vi "Start!.vi"() -> ()   [LabVIEW 2015]
doc: "This VI is designed to launch the VIs needed to do data acquisition on the microscope in the required order. The VIs can be launched from the Glimpse library (used to launch Glimpse itself) or from the plug-ins library (used to launch the data acquisition plug-in and any hardware-control plug-ins that are needed). It is suggested that users modify settings as needed and save the modified version with a name descriptive of the type of experiment. (That's why this is a separate file, not included in the plug-ins library.) (Remember to right-click/Data Operations/Make current value default value so that your altered setting will be saved for the next time!)"
uses:
  h-nu-ixon/Start! globals.vi
  Microscope software version global.vi
  h-nu-ixon/Microscope ID global.vi
  Glimpse core/GLIMPSE Globals.vi
  ixon1024/HAL Camera specifications globals.vi
  h-nu-ixon/knob global.vi
  h-nu-ixon/stage globals.vi
panel:
  out "Header":string
  out "Starting module number:":i16(slide) scale=0.0..10.0
  out "Source":path
  out "Status":string="Ready"
  # "Note:  If this VI is inside an LLB, the above folder names are ignored and the \nLLB name is used instead"
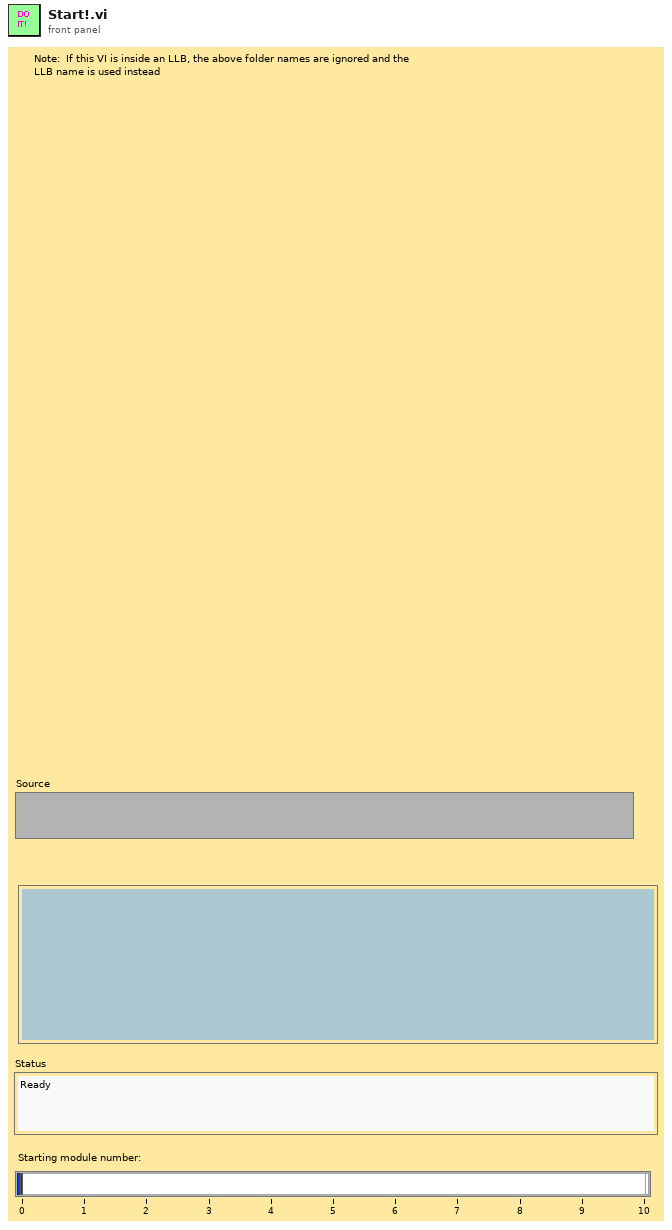
[diagram p1: front panel]
types:
  T1 = cluster{"VI name":string, "Location":enum16{"Plug-ins", "Glimpse"}, "Run":bool, "Minimized?":bool, "Subdirectory (w trailing \"\\\")":string}[]
  T2 = enum32{"Bad", "Idle", "Run top level", "Running"}
  T3 = enum32{"Invalid", "Standard", "Closed", "Hidden", "Minimized", "Maximized"}
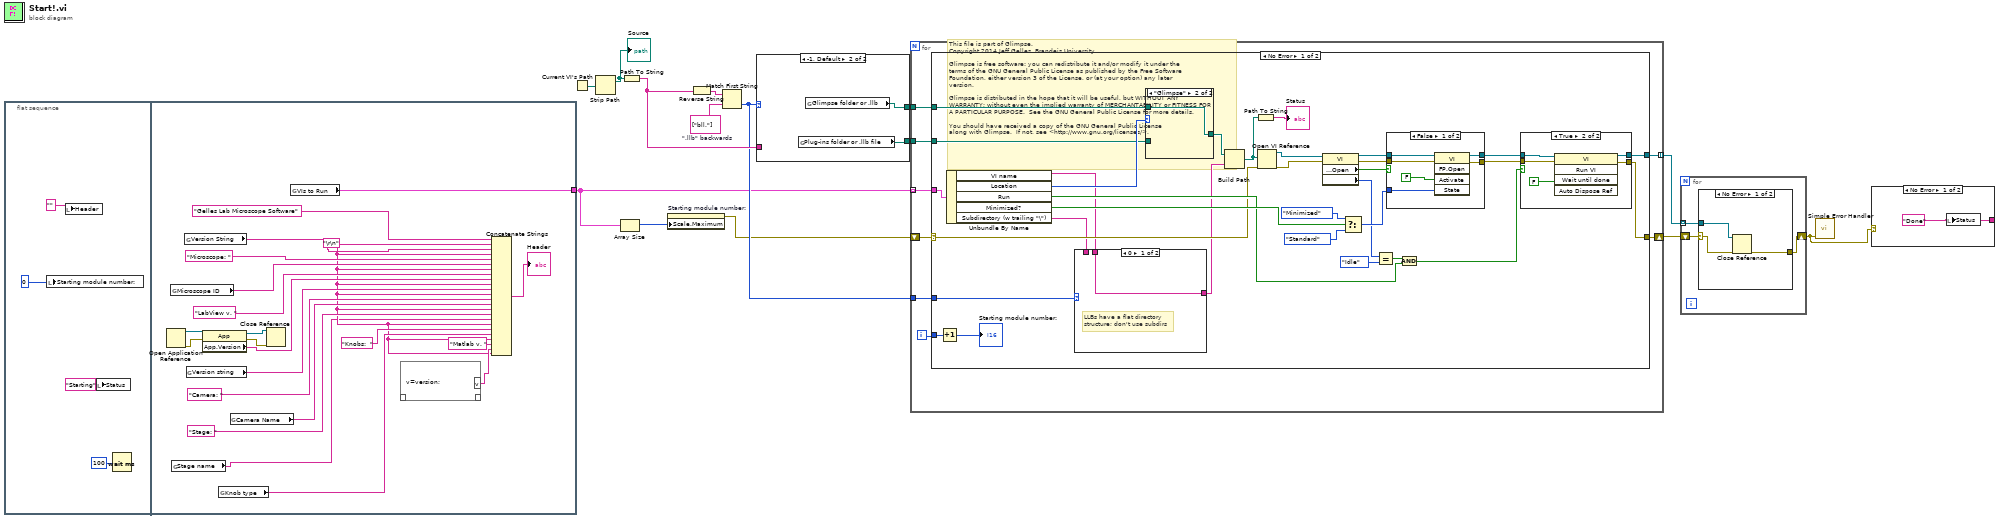
[diagram p0: block diagram]
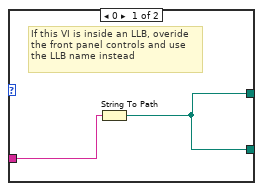
[diagram p2: hidden frame]
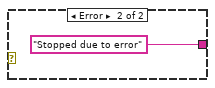
[diagram p3: hidden frame]
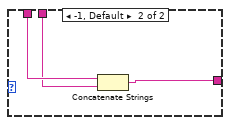
[diagram p5: hidden frame]
diagram:
  w7 = string[] ["bll."]  # ".llb" backwards
  # "This file is part of Glimpse. \nCopyright 2014 Jeff Gelles, Brandeis University.    \n\nGlimpse is free software: you can redistribute it and/or modify it under the \nterms of the GNU General Public License as published by the Free Software \nFoundation, either version 3 of the License, or (at your option) any later \nversion.\n\nGlimpse is distributed in the hope that it will be useful, but WITHOUT ANY \nWARRANTY; without even the implied warranty of MERCHANTABILITY or FITNESS FOR \nA PARTICULAR PURPOSE.  See the GNU General Public License for more details.\n\nYou should have received a copy of the GNU General Public License\nalong with Glimpse.  If not, see <http://www.gnu.org/licenses/>."
  n1 = flat-sequence {
    tunnel: [w23] -> w3
    frame #0 {
      n2 = local write "Starting module number:"(i16 0 ("Module number")) -> ()
      n3 = local write "Header"("" ("Header")) -> ()
      n4 = local write "Status"("Starting" ("Status")) -> ()
      n5 = Wait (ms)(milliseconds to wait=u32 100) -> ()  [unwired: 1 out]
    }
    frame #1 {
      w20 = "\r\n"
      n6 = Open Application Reference() -> (0:w33:errorcluster, 3:w34:refnum<vi>)  [unwired: 1 in, 3 out]
      n7 = global read "Microscope ID global.vi" "Microscope ID"() -> (w36:string)
      n8 = global read "stage globals.vi" "Stage name"() -> (w19:string)
      n9 = global read "Microscope software version global.vi" "Version String"() -> (w38:string)
      n10 = global read "GLIMPSE Globals.vi" "Version string"() -> (w29:string)
      n11 = property class="App"(reference=w34, error in=w33) -> (reference out=w31:refnum<vi>, error out=w32:errorcluster, "App.Version"=w30:string)
      n12 = global read "knob global.vi" "Knob type"() -> (w24:string)
      n13 = global read "HAL Camera specifications globals.vi" "Camera Name"() -> (w27:string)
      n14 = Close Reference(reference=w31, error in (no error)=w32) -> ()  [unwired: 1 out]
      n15 = global read "Start! globals.vi" "VIs to Run"() -> (w23:T1)
      n16 = script code="v=version;"() -> ("v"=w21:string)  [unwired: 1 in, 1 out]
      n17 = Concatenate Strings("Gelles Lab Microscope Software" ("string"), w20, w38, w20, "Microscope: " ("string"), w36, w20, "LabView v. " ("string"), w30, w20, w29, w20, "Camera: " ("string"), w27, w20, "Stage: " ("string"), w19, w20, "Knobs:  " ("string"), w24, w20, "Matlab v. " ("string"), w21, w20) -> (→"Header":string)
    }
  }
  n18 = Current VI's Path() -> (path=w9:path)
  n19 = Strip Path(path=w9) -> (stripped path=w6:path)  [unwired: 1 out]
  "Source" <- w6
  n20 = Array Size(array=w3) -> (size(s)=w2:i32)
  n21 = Path To String(path=w6) -> (string=w5:string)
  n22 = property on="Starting module number:" class="Slide (strict)"("Scale.Maximum"=w2) -> (error out=w1:errorcluster)  [unwired: 2 in, 1 out]
  n23 = Reverse String(1:w5) -> (0:w8:string)
  n24 = Match First String(2:w7, 3:w8) -> (0:w4:i32)  [unwired: 1 out]
  n25 = case shown="-1, Default" w4 {
    tunnel: [w42 w43] -> w14
    tunnel: [w42 w44] -> w13
    tunnel: w5 -> [w41 _]
    frame 0 {
      # "If this VI is inside an LLB, overide\nthe front panel controls and use\nthe LLB name instead"
      n26 = String To Path(string=w41) -> (path=w42:path)
    }
    frame -1, Default {
      n27 = global read "Start! globals.vi" "Plug-ins folder or .llb file"() -> (w44:path)
      n28 = global read "Start! globals.vi" "Glimpse folder or .llb"() -> (w43:path)
    }
  }
  n29 = for {
    tunnel: w3 -> [w52] mode=indexing
    tunnel: w14 -> [w51]
    tunnel: w13 -> [w50]
    shift-right: [w49] -> w12
    shift-left: w1 -> [w48]
    tunnel: [w47] -> w11 mode=indexing
    tunnel: w4 -> [w46]
    i -> [w45]
    n30 = case shown="No Error" w48 {
      selector: w48 -> [w62 w106]
      tunnel: w52 -> [w81 _]
      tunnel: w51 -> [w78 _]
      tunnel: w50 -> [w77 _]
      tunnel: [w61 w106] -> w49
      tunnel: [w60 _] -> w47
      tunnel: w46 -> [w58 _]
      tunnel: w45 -> [w54 _]
      frame No Error {
        n31 = Increment(x=w54) -> (x+1=→"Starting module number:":i32)
        n32 = Unbundle By Name(w81) -> ("VI name"=w56:string, "Location"=w80:enum16{"Plug-ins", "Glimpse"}, "Run"=w66:bool, "Minimized?"=w71:bool, "Subdirectory (w trailing \"\\\")"=w57:string)
        n33 = case shown="0" w58 {
          tunnel: w57 -> [_ w88]
          tunnel: w56 -> [w85 w87]
          tunnel: [w85 w86] -> w55
          frame 0 {
            # "LLBs have a flat directory\nstructure; don't use subdirs"
          }
          frame -1, Default {
            n34 = Concatenate Strings(w88, w87) -> (w86:string)
          }
        }
        n35 = case shown="\"Glimpse\"" w80 {
          tunnel: [w96 w97] -> w79
          tunnel: w78 -> [_ w97]
          tunnel: w77 -> [w96 _]
          frame "Plug-ins", Default {
          }
          frame "Glimpse" {
          }
        }
        n36 = Build Path(base path=w79, name or relative path=w55) -> (appended path=w76:path)
        n37 = Path To String(path=w76) -> (string=→"Status":string)
        n38 = Open VI Reference(vi path=w76, error in (no error)=w62) -> (vi reference=w74:refnum<vi>, error out=w75:errorcluster)  [unwired: 4 out]
        n39 = property class="VI"(reference=w74, error in=w75) -> (reference out=w83:refnum<vi>, error out=w84:errorcluster, "Front Panel Window:Open"=w82:bool, "Execution:State"=w69:T2)
        n40 = Select(t=T3."Minimized" ("State"), s=w71, f=T3."Standard" ("State")) -> (s? t:f=w70:T3)
        n41 = Equal?(x=w69, y=T2."Idle") -> (x = y?=w67:bool)
        n42 = case shown="False" w82 {
          tunnel: w83 -> [w99 w105]
          tunnel: [w102 w105] -> w65
          tunnel: [w101 w104] -> w64
          tunnel: w84 -> [w100 w104]
          tunnel: w70 -> [w98 _]
          frame False {
            n43 = invoke class="VI" method="FP.Open"(reference=w99, error in=w100, "Activate"=FALSE, "State"=w98) -> (reference out=w102:refnum<vi>, error out=w101:errorcluster)  [unwired: 1 in, 3 out]
          }
          frame True {
          }
        }
        n44 = And(x=w67, y=w66) -> (x .and. y?=w63:bool)
        n45 = case shown="True" w63 {
          tunnel: w65 -> [w90 w91]
          tunnel: [w90 w94] -> w60
          tunnel: [w89 w93] -> w61
          tunnel: w64 -> [w89 w92]
          frame False {
          }
          frame True {
            n46 = invoke class="VI" method="Run VI"(reference=w91, error in=w92, "Wait until done"=FALSE ("Activate")) -> (reference out=w94:refnum<vi>, error out=w93:errorcluster)  [unwired: 2 in, 3 out]
          }
        }
      }
      frame Error {
      }
    }
  }
  n47 = for {
    tunnel: w11 -> [w108] mode=indexing
    shift-right: [w107] -> w10
    shift-left: w12 -> [w109]
    n48 = case shown="No Error" w109 {
      selector: w109 -> [w111 w113]
      tunnel: w108 -> [w112 _]
      tunnel: [w110 w113] -> w107
      frame No Error {
        n49 = Close Reference(reference=w112, error in (no error)=w111) -> (error out=w110:errorcluster)
      }
      frame Error {
      }
    }
  }
  n50 = call <vilib>:"Simple Error Handler.vi"("error in (no error)"=w10) -> ()  [unwired: 1 in, 8 out]
  n51 = case shown="No Error" w10 {
    tunnel: [w114 "Stopped due to error" ("Status")] -> _
    frame No Error {
      w114 = "Done" ("Status")
      n52 = local write "Status"(w114) -> ()
    }
    frame Error {
    }
  }
